vi "golpi_struct_assign_test.vi"() -> (0 "error out":errorcluster)   [LabVIEW 2013, in "GOLPI library.lvlib"]
uses:
  GOLPI library.lvlib
  Struct Item Record.ctl
  Struct Item Types.ctl
panel:
  out "struct items":T1[](array[typedef])
  out "element":T1
  in  "Cluster":T3
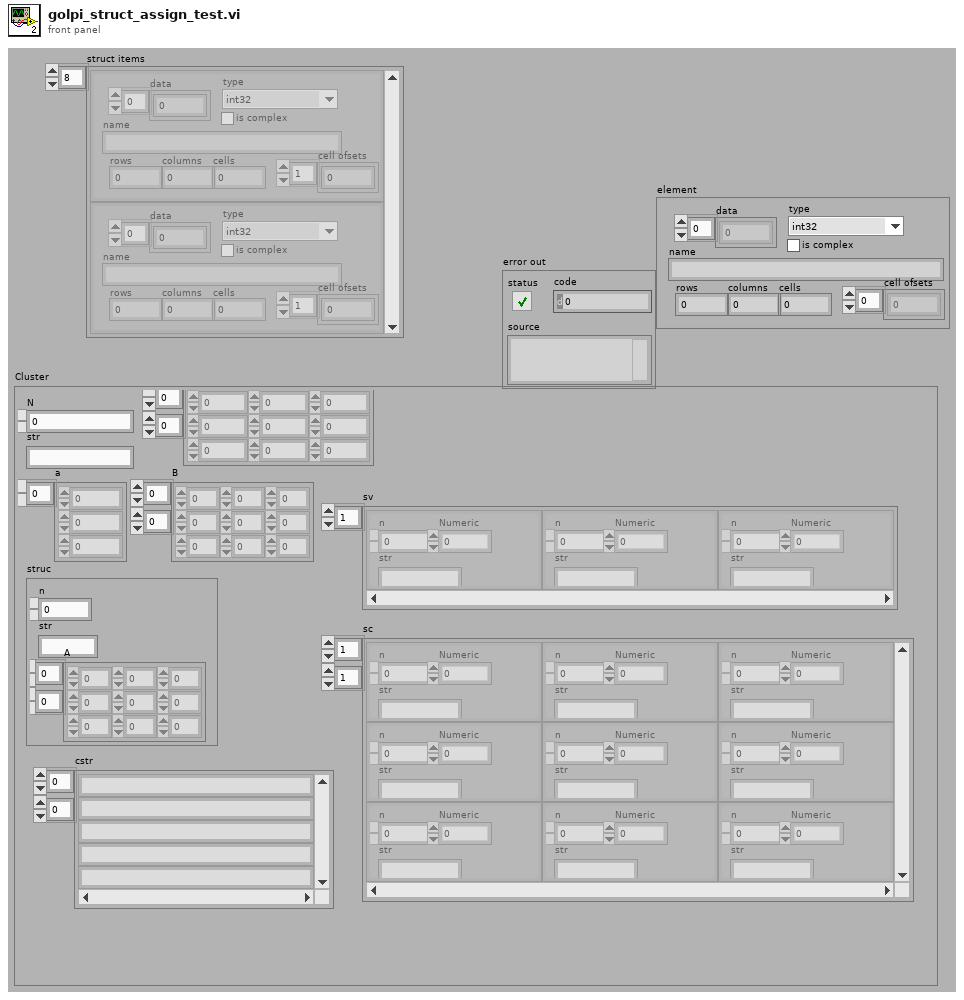
[diagram p1: front panel]
types:
  T1 = typedef "GOLPI library.lvlib/Struct Item Record.ctl" = cluster{"data":u8[], "type":T2, "name":string, "rows":i32, "columns":i32, "cells":i32, "is complex":bool, "cell ofsets":u32[]}
  T2 = typedef "GOLPI library.lvlib/Struct Item Types.ctl" = enum16{"int32", "uint32", "single", "double", "string", "cell array"}
  T3 = cluster{"N":dbl, "str":string, "a":dbl[], "struc":cluster{"n":dbl, "str":string, "A":dbl[][]}, "B":dbl[][], "ca":cdb[][], "sv":cluster{"n":dbl, "str":string, "Numeric":cdb}[], "sc":cluster{"n":dbl, "str":string, "Numeric":cdb}[][], "cstr":string[][]}
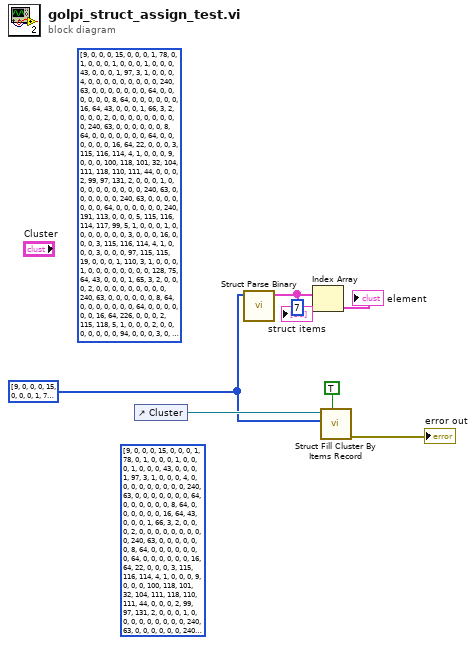
[diagram p0: block diagram]
diagram:
  w1 = u8[] [9, 0, 0, 0, 15, 0, 0, 0, 1, 78, 0, 1, 0, 0, 0, 1, 0, 0, 0, 1, 0, 0, 0, 43, 0, 0, 0, 1, 97, 3, 1, 0, 0, 0, 4, 0, 0, 0, 0, 0, 0, 0, 0, 0, 240, 63, 0, 0, 0, 0, 0, 0, 0, 64, 0, 0, 0, 0, 0, 0, 8, 64, 0, 0, 0, 0, 0, 0, 16, 64, 43, 0, 0, 0, 1, 66, 3, 2, 0, 0, 0, 2, 0, 0, 0, 0, 0, 0, 0, 0, 0, 240, 63, 0, 0, 0, 0, 0, 0, 8, 64, 0, 0, 0, 0, 0, 0, 0, 64, 0, 0, 0, 0, 0, 0, 16, 64, 22, 0, 0, 0, 3, 115, 116, 114, 4, 1, 0, 0, 0, 9, 0, 0, 0, 100, 118, 101, 32, 104, 111, 118, 110, 111, 44, 0, 0, 0, 2, 99, 97, 131, 2, 0, 0, 0, 1, 0, 0, 0, 0, 0, 0, 0, 0, 0, 240, 63, 0, 0, 0, 0, 0, 0, 240, 63, 0, 0, 0, 0, 0, 0, 0, 64, 0, 0, 0, 0, 0, 0, 240, 191, 113, 0, 0, 0, 5, 115, 116, 114, 117, 99, 5, 1, 0, 0, 0, 1, 0, 0, 0, 0, 0, 0, 0, 3, 0, 0, 0, 16, 0, 0, 0, 3, 115, 116, 114, 4, 1, 0, 0, 0, 3, 0, 0, 0, 97, 115, 115, 19, 0, 0, 0, 1, 110, 3, 1, 0, 0, 0, 1, 0, 0, 0, 0, 0, 0, 0, 0, 128, 75, 64, 43, 0, 0, 0, 1, 65, 3, 2, 0, 0, 0, 2, 0, 0, 0, 0, 0, 0, 0, 0, 0, 240, 63, 0, 0, 0, 0, 0, 0, 8, 64, 0, 0, 0, 0, 0, 0, 0, 64, 0, 0, 0, 0, 0, 0, 16, 64, 226, 0, 0, 0, 2, 115, 118, 5, 1, 0, 0, 0, 2, 0, 0, 0, 0, 0, 0, 0, 94, 0, 0, 0, 3, 0, 0, 0, 16, 0, 0, 0, 3, 115, 116, 114, 4, 1, 0, 0, 0, 3, 0, 0, 0, 97, 115, 115, 19, 0, 0, 0, 1, 110, 3, 1, 0, 0, 0, 1, 0, 0, 0, 0, 0, 0, 0, 0, 128, 75, 64, 43, 0, 0, 0, 1, 65, 3, 2, 0, 0, 0, 2, 0, 0, 0, 0, 0, 0, 0, 0, 0, 240, 63, 0, 0, 0, 0, 0, 0, 8, 64, 0, 0, 0, 0, 0, 0, 0, 64, 0, 0, 0, 0, 0, 0, 16, 64, 3, 0, 0, 0, 34, 0, 0, 0, 3, 115, 116, 114, 4, 1, 0, 0, 0, 21, 0, 0, 0, 110, 101, 106, 97, 107, 101, 106, 32, 106, 105, 110, 101, 106, 32, 114, 101, 116, 101, 122, 101, 99, 19, 0, 0, 0, 1, 110, 3, 1, 0, 0, 0, 1, 0, 0, 0, 0, 0, 0, 0, 0, 0, 86, 64, 43, 0, 0, 0, 1, 65, 3, 2, 0, 0, 0, 2, 0, 0, 0, 0, 0, 0, 0, 0, 0, 240, 63, 0, 0, 0, 0, 0, 0, 8, 64, 0, 0, 0, 0, 0, 0, 0, 64, 0, 0, 0, 0, 0, 0, 16, 64, 148, 1, 0, 0, 2, 115, 99, 5, 2, 0, 0, 0, 2, 0, 0, 0, 0, 0, 0, 0, 94, 0, 0, 0, 188, 0, 0, 0, 26, 1, 0, 0, 3, 0, 0, 0, 16, 0, 0, 0, 3, 115, 116, 114, 4, 1, 0, 0, 0, 3, 0, 0, 0, 97, 115, 115, 19, 0, 0, 0, 1, 110, 3, 1, 0, 0, 0, 1, 0, 0, 0, 0, 0, 0, 0, 0, 128, 75, 64, 43, 0, 0, 0, 1, 65, 3, 2, 0, 0, 0, 2, 0, 0, 0, 0, 0, 0, 0, 0, 0, 240, 63, 0, 0, 0, 0, 0, 0, 8, 64, 0, 0, 0, 0, 0, 0, 0, 64, 0, 0, 0, 0, 0, 0, 16, 64, 3, 0, 0, 0, 16, 0, 0, 0, 3, 115, 116, 114, 4, 1, 0, 0, 0, 3, 0, 0, 0, 97, 115, 115, 19, 0, 0, 0, 1, 110, 3, 1, 0, 0, 0, 1, 0, 0, 0, 0, 0, 0, 0, 0, 128, 75, 64, 43, 0, 0, 0, 1, 65, 3, 2, 0, 0, 0, 2, 0, 0, 0, 0, 0, 0, 0, 0, 0, 240, 63, 0, 0, 0, 0, 0, 0, 8, 64, 0, 0, 0, 0, 0, 0, 0, 64, 0, 0, 0, 0, 0, 0, 16, 64, 3, 0, 0, 0, 16, 0, 0, 0, 3, 115, 116, 114, 4, 1, 0, 0, 0, 3, 0, 0, 0, 97, 115, 115, 19, 0, 0, 0, 1, 110, 3, 1, 0, 0, 0, 1, 0, 0, 0, 0, 0, 0, 0, 0, 128, 75, 64, 43, 0, 0, 0, 1, 65, 3, 2, 0, 0, 0, 2, 0, 0, 0, 0, 0, 0, 0, 0, 0, 240, 63, 0, 0, 0, 0, 0, 0, 8, 64, 0, 0, 0, 0, 0, 0, 0, 64, 0, 0, 0, 0, 0, 0, 16, 64, 3, 0, 0, 0, 16, 0, 0, 0, 3, 115, 116, 114, 4, 1, 0, 0, 0, 3, 0, 0, 0, 97, 115, 115, 19, 0, 0, 0, 1, 110, 3, 1, 0, 0, 0, 1, 0, 0, 0, 0, 0, 0, 0, 0, 128, 75, 64, 43, 0, 0, 0, 1, 65, 3, 2, 0, 0, 0, 2, 0, 0, 0, 0, 0, 0, 0, 0, 0, 240, 63, 0, 0, 0, 0, 0, 0, 8, 64, 0, 0, 0, 0, 0, 0, 0, 64, 0, 0, 0, 0, 0, 0, 16, 64, 128, 0, 0, 0, 4, 99, 115, 116, 114, 5, 1, 0, 0, 0, 3, 0, 0, 0, 0, 0, 0, 0, 23, 0, 0, 0, 51, 0, 0, 0, 1, 0, 0, 0, 15, 0, 0, 0, 0, 4, 1, 0, 0, 0, 5, 0, 0, 0, 115, 108, 111, 118, 111, 1, 0, 0, 0, 20, 0, 0, 0, 0, 4, 1, 0, 0, 0, 10, 0, 0, 0, 106, 105, 110, 121, 32, 115, 108, 111, 118, 111, 1, 0, 0, 0, 43, 0, 0, 0, 0, 4, 1, 0, 0, 0, 33, 0, 0, 0, 78, 101, 106, 97, 107, 97, 32, 106, 97, 107, 111, 122, 101, 32, 118, 101, 116, 97, 32, 110, 101, 98, 111, 32, 116, 97, 107, 32, 110, 101, 99, 111, 46] ("unsigned 8bit integer")
  (unwired) u8[] [9, 0, 0, 0, 15, 0, 0, 0, 1, 78, 0, 1, 0, 0, 0, 1, 0, 0, 0, 1, 0, 0, 0, 43, 0, 0, 0, 1, 97, 3, 1, 0, 0, 0, 4, 0, 0, 0, 0, 0, 0, 0, 0, 0, 240, 63, 0, 0, 0, 0, 0, 0, 0, 64, 0, 0, 0, 0, 0, 0, 8, 64, 0, 0, 0, 0, 0, 0, 16, 64, 43, 0, 0, 0, 1, 66, 3, 2, 0, 0, 0, 2, 0, 0, 0, 0, 0, 0, 0, 0, 0, 240, 63, 0, 0, 0, 0, 0, 0, 8, 64, 0, 0, 0, 0, 0, 0, 0, 64, 0, 0, 0, 0, 0, 0, 16, 64, 22, 0, 0, 0, 3, 115, 116, 114, 4, 1, 0, 0, 0, 9, 0, 0, 0, 100, 118, 101, 32, 104, 111, 118, 110, 111, 44, 0, 0, 0, 2, 99, 97, 131, 2, 0, 0, 0, 1, 0, 0, 0, 0, 0, 0, 0, 0, 0, 240, 63, 0, 0, 0, 0, 0, 0, 240, 63, 0, 0, 0, 0, 0, 0, 0, 64, 0, 0, 0, 0, 0, 0, 240, 191, 113, 0, 0, 0, 5, 115, 116, 114, 117, 99, 5, 1, 0, 0, 0, 1, 0, 0, 0, 0, 0, 0, 0, 3, 0, 0, 0, 16, 0, 0, 0, 3, 115, 116, 114, 4, 1, 0, 0, 0, 3, 0, 0, 0, 97, 115, 115, 19, 0, 0, 0, 1, 110, 3, 1, 0, 0, 0, 1, 0, 0, 0, 0, 0, 0, 0, 0, 128, 75, 64, 43, 0, 0, 0, 1, 65, 3, 2, 0, 0, 0, 2, 0, 0, 0, 0, 0, 0, 0, 0, 0, 240, 63, 0, 0, 0, 0, 0, 0, 8, 64, 0, 0, 0, 0, 0, 0, 0, 64, 0, 0, 0, 0, 0, 0, 16, 64, 226, 0, 0, 0, 2, 115, 118, 5, 1, 0, 0, 0, 2, 0, 0, 0, 0, 0, 0, 0, 94, 0, 0, 0, 3, 0, 0, 0, 16, 0, 0, 0, 3, 115, 116, 114, 4, 1, 0, 0, 0, 3, 0, 0, 0, 97, 115, 115, 19, 0, 0, 0, 1, 110, 3, 1, 0, 0, 0, 1, 0, 0, 0, 0, 0, 0, 0, 0, 128, 75, 64, 43, 0, 0, 0, 1, 65, 3, 2, 0, 0, 0, 2, 0, 0, 0, 0, 0, 0, 0, 0, 0, 240, 63, 0, 0, 0, 0, 0, 0, 8, 64, 0, 0, 0, 0, 0, 0, 0, 64, 0, 0, 0, 0, 0, 0, 16, 64, 3, 0, 0, 0, 34, 0, 0, 0, 3, 115, 116, 114, 4, 1, 0, 0, 0, 21, 0, 0, 0, 110, 101, 106, 97, 107, 101, 106, 32, 106, 105, 110, 101, 106, 32, 114, 101, 116, 101, 122, 101, 99, 19, 0, 0, 0, 1, 110, 3, 1, 0, 0, 0, 1, 0, 0, 0, 0, 0, 0, 0, 0, 0, 86, 64, 43, 0, 0, 0, 1, 65, 3, 2, 0, 0, 0, 2, 0, 0, 0, 0, 0, 0, 0, 0, 0, 240, 63, 0, 0, 0, 0, 0, 0, 8, 64, 0, 0, 0, 0, 0, 0, 0, 64, 0, 0, 0, 0, 0, 0, 16, 64, 148, 1, 0, 0, 2, 115, 99, 5, 2, 0, 0, 0, 2, 0, 0, 0, 0, 0, 0, 0, 94, 0, 0, 0, 188, 0, 0, 0, 26, 1, 0, 0, 3, 0, 0, 0, 16, 0, 0, 0, 3, 115, 116, 114, 4, 1, 0, 0, 0, 3, 0, 0, 0, 97, 115, 115, 19, 0, 0, 0, 1, 110, 3, 1, 0, 0, 0, 1, 0, 0, 0, 0, 0, 0, 0, 0, 128, 75, 64, 43, 0, 0, 0, 1, 65, 3, 2, 0, 0, 0, 2, 0, 0, 0, 0, 0, 0, 0, 0, 0, 240, 63, 0, 0, 0, 0, 0, 0, 8, 64, 0, 0, 0, 0, 0, 0, 0, 64, 0, 0, 0, 0, 0, 0, 16, 64, 3, 0, 0, 0, 16, 0, 0, 0, 3, 115, 116, 114, 4, 1, 0, 0, 0, 3, 0, 0, 0, 97, 115, 115, 19, 0, 0, 0, 1, 110, 3, 1, 0, 0, 0, 1, 0, 0, 0, 0, 0, 0, 0, 0, 128, 75, 64, 43, 0, 0, 0, 1, 65, 3, 2, 0, 0, 0, 2, 0, 0, 0, 0, 0, 0, 0, 0, 0, 240, 63, 0, 0, 0, 0, 0, 0, 8, 64, 0, 0, 0, 0, 0, 0, 0, 64, 0, 0, 0, 0, 0, 0, 16, 64, 3, 0, 0, 0, 16, 0, 0, 0, 3, 115, 116, 114, 4, 1, 0, 0, 0, 3, 0, 0, 0, 97, 115, 115, 19, 0, 0, 0, 1, 110, 3, 1, 0, 0, 0, 1, 0, 0, 0, 0, 0, 0, 0, 0, 128, 75, 64, 43, 0, 0, 0, 1, 65, 3, 2, 0, 0, 0, 2, 0, 0, 0, 0, 0, 0, 0, 0, 0, 240, 63, 0, 0, 0, 0, 0, 0, 8, 64, 0, 0, 0, 0, 0, 0, 0, 64, 0, 0, 0, 0, 0, 0, 16, 64, 3, 0, 0, 0, 16, 0, 0, 0, 3, 115, 116, 114, 4, 1, 0, 0, 0, 3, 0, 0, 0, 97, 115, 115, 19, 0, 0, 0, 1, 110, 3, 1, 0, 0, 0, 1, 0, 0, 0, 0, 0, 0, 0, 0, 128, 75, 64, 43, 0, 0, 0, 1, 65, 3, 2, 0, 0, 0, 2, 0, 0, 0, 0, 0, 0, 0, 0, 0, 240, 63, 0, 0, 0, 0, 0, 0, 8, 64, 0, 0, 0, 0, 0, 0, 0, 64, 0, 0, 0, 0, 0, 0, 16, 64, 128, 0, 0, 0, 4, 99, 115, 116, 114, 5, 1, 0, 0, 0, 3, 0, 0, 0, 0, 0, 0, 0, 23, 0, 0, 0, 51, 0, 0, 0, 1, 0, 0, 0, 15, 0, 0, 0, 0, 4, 1, 0, 0, 0, 5, 0, 0, 0, 115, 108, 111, 118, 111, 1, 0, 0, 0, 20, 0, 0, 0, 0, 4, 1, 0, 0, 0, 10, 0, 0, 0, 106, 105, 110, 121, 32, 115, 108, 111, 118, 111, 1, 0, 0, 0, 43, 0, 0, 0, 0, 4, 1, 0, 0, 0, 33, 0, 0, 0, 78, 101, 106, 97, 107, 97, 32, 106, 97, 107, 111, 122, 101, 32, 118, 101, 116, 97, 32, 110, 101, 98, 111, 32, 116, 97, 107, 32, 110, 101, 99, 111, 46] ("unsigned 8bit integer")
  (unwired) u8[] [9, 0, 0, 0, 15, 0, 0, 0, 1, 78, 0, 1, 0, 0, 0, 1, 0, 0, 0, 1, 0, 0, 0, 43, 0, 0, 0, 1, 97, 3, 1, 0, 0, 0, 4, 0, 0, 0, 0, 0, 0, 0, 0, 0, 240, 63, 0, 0, 0, 0, 0, 0, 0, 64, 0, 0, 0, 0, 0, 0, 8, 64, 0, 0, 0, 0, 0, 0, 16, 64, 43, 0, 0, 0, 1, 66, 3, 2, 0, 0, 0, 2, 0, 0, 0, 0, 0, 0, 0, 0, 0, 240, 63, 0, 0, 0, 0, 0, 0, 8, 64, 0, 0, 0, 0, 0, 0, 0, 64, 0, 0, 0, 0, 0, 0, 16, 64, 22, 0, 0, 0, 3, 115, 116, 114, 4, 1, 0, 0, 0, 9, 0, 0, 0, 100, 118, 101, 32, 104, 111, 118, 110, 111, 44, 0, 0, 0, 2, 99, 97, 131, 2, 0, 0, 0, 1, 0, 0, 0, 0, 0, 0, 0, 0, 0, 240, 63, 0, 0, 0, 0, 0, 0, 240, 63, 0, 0, 0, 0, 0, 0, 0, 64, 0, 0, 0, 0, 0, 0, 240, 191, 113, 0, 0, 0, 5, 115, 116, 114, 117, 99, 5, 1, 0, 0, 0, 1, 0, 0, 0, 0, 0, 0, 0, 3, 0, 0, 0, 16, 0, 0, 0, 3, 115, 116, 114, 4, 1, 0, 0, 0, 3, 0, 0, 0, 97, 115, 115, 19, 0, 0, 0, 1, 110, 3, 1, 0, 0, 0, 1, 0, 0, 0, 0, 0, 0, 0, 0, 128, 75, 64, 43, 0, 0, 0, 1, 65, 3, 2, 0, 0, 0, 2, 0, 0, 0, 0, 0, 0, 0, 0, 0, 240, 63, 0, 0, 0, 0, 0, 0, 8, 64, 0, 0, 0, 0, 0, 0, 0, 64, 0, 0, 0, 0, 0, 0, 16, 64, 226, 0, 0, 0, 2, 115, 118, 5, 1, 0, 0, 0, 2, 0, 0, 0, 0, 0, 0, 0, 94, 0, 0, 0, 3, 0, 0, 0, 16, 0, 0, 0, 3, 115, 116, 114, 4, 1, 0, 0, 0, 3, 0, 0, 0, 97, 115, 115, 19, 0, 0, 0, 1, 110, 3, 1, 0, 0, 0, 1, 0, 0, 0, 0, 0, 0, 0, 0, 128, 75, 64, 43, 0, 0, 0, 1, 65, 3, 2, 0, 0, 0, 2, 0, 0, 0, 0, 0, 0, 0, 0, 0, 240, 63, 0, 0, 0, 0, 0, 0, 8, 64, 0, 0, 0, 0, 0, 0, 0, 64, 0, 0, 0, 0, 0, 0, 16, 64, 3, 0, 0, 0, 34, 0, 0, 0, 3, 115, 116, 114, 4, 1, 0, 0, 0, 21, 0, 0, 0, 110, 101, 106, 97, 107, 101, 106, 32, 106, 105, 110, 101, 106, 32, 114, 101, 116, 101, 122, 101, 99, 19, 0, 0, 0, 1, 110, 3, 1, 0, 0, 0, 1, 0, 0, 0, 0, 0, 0, 0, 0, 0, 86, 64, 43, 0, 0, 0, 1, 65, 3, 2, 0, 0, 0, 2, 0, 0, 0, 0, 0, 0, 0, 0, 0, 240, 63, 0, 0, 0, 0, 0, 0, 8, 64, 0, 0, 0, 0, 0, 0, 0, 64, 0, 0, 0, 0, 0, 0, 16, 64, 148, 1, 0, 0, 2, 115, 99, 5, 2, 0, 0, 0, 2, 0, 0, 0, 0, 0, 0, 0, 94, 0, 0, 0, 188, 0, 0, 0, 26, 1, 0, 0, 3, 0, 0, 0, 16, 0, 0, 0, 3, 115, 116, 114, 4, 1, 0, 0, 0, 3, 0, 0, 0, 97, 115, 115, 19, 0, 0, 0, 1, 110, 3, 1, 0, 0, 0, 1, 0, 0, 0, 0, 0, 0, 0, 0, 128, 75, 64, 43, 0, 0, 0, 1, 65, 3, 2, 0, 0, 0, 2, 0, 0, 0, 0, 0, 0, 0, 0, 0, 240, 63, 0, 0, 0, 0, 0, 0, 8, 64, 0, 0, 0, 0, 0, 0, 0, 64, 0, 0, 0, 0, 0, 0, 16, 64, 3, 0, 0, 0, 16, 0, 0, 0, 3, 115, 116, 114, 4, 1, 0, 0, 0, 3, 0, 0, 0, 97, 115, 115, 19, 0, 0, 0, 1, 110, 3, 1, 0, 0, 0, 1, 0, 0, 0, 0, 0, 0, 0, 0, 128, 75, 64, 43, 0, 0, 0, 1, 65, 3, 2, 0, 0, 0, 2, 0, 0, 0, 0, 0, 0, 0, 0, 0, 240, 63, 0, 0, 0, 0, 0, 0, 8, 64, 0, 0, 0, 0, 0, 0, 0, 64, 0, 0, 0, 0, 0, 0, 16, 64, 3, 0, 0, 0, 16, 0, 0, 0, 3, 115, 116, 114, 4, 1, 0, 0, 0, 3, 0, 0, 0, 97, 115, 115, 19, 0, 0, 0, 1, 110, 3, 1, 0, 0, 0, 1, 0, 0, 0, 0, 0, 0, 0, 0, 128, 75, 64, 43, 0, 0, 0, 1, 65, 3, 2, 0, 0, 0, 2, 0, 0, 0, 0, 0, 0, 0, 0, 0, 240, 63, 0, 0, 0, 0, 0, 0, 8, 64, 0, 0, 0, 0, 0, 0, 0, 64, 0, 0, 0, 0, 0, 0, 16, 64, 3, 0, 0, 0, 16, 0, 0, 0, 3, 115, 116, 114, 4, 1, 0, 0, 0, 3, 0, 0, 0, 97, 115, 115, 19, 0, 0, 0, 1, 110, 3, 1, 0, 0, 0, 1, 0, 0, 0, 0, 0, 0, 0, 0, 128, 75, 64, 43, 0, 0, 0, 1, 65, 3, 2, 0, 0, 0, 2, 0, 0, 0, 0, 0, 0, 0, 0, 0, 240, 63, 0, 0, 0, 0, 0, 0, 8, 64, 0, 0, 0, 0, 0, 0, 0, 64, 0, 0, 0, 0, 0, 0, 16, 64, 38, 0, 0, 0, 4, 99, 115, 116, 114, 5, 1, 0, 0, 0, 3, 0, 0, 0, 0, 0, 0, 0, 4, 0, 0, 0, 8, 0, 0, 0, 0, 0, 0, 0, 0, 0, 0, 0, 0, 0, 0, 0] ("data in")
  n1 = control-ref of="Cluster"() -> (w5:refnum<vi>)
  n2 = call "Struct Parse Binary.vi"("data in"=w1) -> ("struct items"=w4:T1[])  [unwired: 9 in, 1 out]
  "struct items" <- w4
  n3 = Index Array(array=w4, index=7) -> (element=→"element":T1)
  n4 = call "Struct Fill Cluster By Items Record.vi"("reinit cluster to default (false)"=TRUE, "data in"=w1, "cluster ref (empty)"=w5) -> ("error out"=→"error out":errorcluster)  [unwired: 6 in, 2 out]
